vi "CMD_FITLINE.vi"(8 "error in (no error)":errorcluster, 10 "Arguments":string[](array[string]), 11 "gScript Interpreter in":refnum<class "gScript Interpreter.lvclass">) -> (0 "error out":errorcluster, 3 "gScript Interpreter out":refnum<class "gScript Interpreter.lvclass">)   [LabVIEW 2022 SP3, in "gScript Interpreter.lvclass"]
uses:
  gScript Interpreter.lvclass
  gScript Interpreter.lvclass/gScript Interpreter.ctl
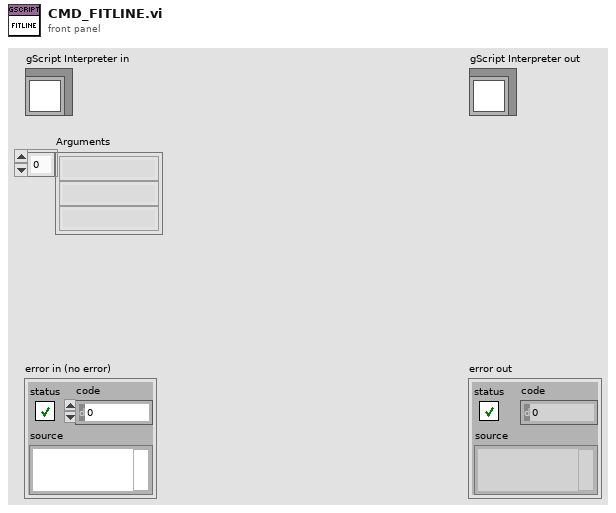
[diagram p1: front panel]
types:
  T1 = typedef "Memory Cell.ctl" = cluster{"type":T2, "x":dbl, "y":dbl, "z":dbl, "w":dbl}
  T2 = typedef "Memory Cell Type Enum.ctl" = enum16{"integer", "float", "vector", "rotation"}
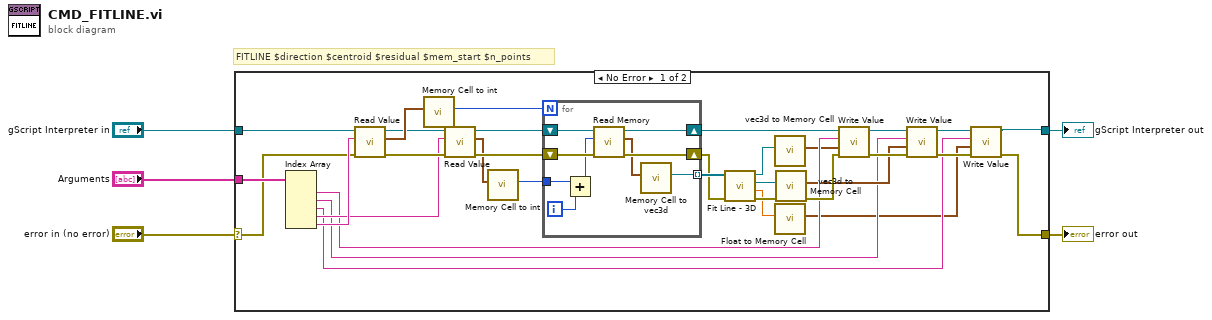
[diagram p0: block diagram]
diagram:
  # "FITLINE $direction $centroid $residual $mem_start $n_points"
  n1 = case shown="No Error" "error in (no error)" {
    selector: "error in (no error)" -> [w34 w48]
    tunnel: [w6 w48] -> w4
    tunnel: [w7 w47] -> w2
    tunnel: "gScript Interpreter in" -> [w36 w47]
    tunnel: "Arguments" -> [w37 _]
    frame No Error {
      n2 = Index Array(array=w37) -> (element #1=w14:string, element #2=w11:string, element #3=w10:string, element #4=w29:string, element #5=w35:string)  [unwired: 5 in]
      n3 = call-dynamic "Read Value.vi"("error in (no error)"=w34, "String in"=w35, "gScript Interpreter in"=w36) -> ("error out"=w30:errorcluster, "Memory Cell"=w33:T1, "gScript Interpreter out"=w31:refnum<class "gScript Interpreter.lvclass">)  [unwired: 6 in]
      n4 = call "Memory Cell to int.vi"("Memory Cell"=w33) -> ("Int out"=w32:i32)  [unwired: 10 in]
      n5 = call-dynamic "Read Value.vi"("error in (no error)"=w30, "String in"=w29, "gScript Interpreter in"=w31) -> ("error out"=w27:errorcluster, "Memory Cell"=w26:T1, "gScript Interpreter out"=w28:refnum<class "gScript Interpreter.lvclass">)  [unwired: 6 in]
      n6 = call "Memory Cell to int.vi"("Memory Cell"=w26) -> ("Int out"=w25:i32)  [unwired: 10 in]
      n7 = for {
        N: w32 -> [_]
        shift-right: [w45] -> w22
        shift-left: w28 -> [w46]
        shift-right: [w43] -> w23
        shift-left: w27 -> [w44]
        tunnel: [w41] -> w24 mode=indexing
        tunnel: w25 -> [w39]
        i -> [w40]
        n8 = Add(x=w39, y=w40) -> (x+y=w38:i32)
        n9 = call-dynamic "Read Memory.vi"("error in (no error)"=w44, "Memory Address"=w38, "gScript Interpreter in"=w46) -> ("error out"=w43:errorcluster, "Memory Cell"=w42:T1, "gScript Interpreter out"=w45:refnum<class "gScript Interpreter.lvclass">)  [unwired: 6 in]
        n10 = call "Memory Cell to vec3d.vi"("Memory Cell"=w42) -> ("Vec3d out"=w41:refnum<class "Vec3d.lvclass">)  [unwired: 10 in]
      }
      n11 = call "Fit Line - 3D.vi"("error in (no error)"=w23, "Points"=w24) -> ("error out"=w19:errorcluster, "residual"=w9:dbl, "centroid"=w15:refnum<class "Vec3d.lvclass">, "direction"=w16:refnum<class "Vec3d.lvclass">)  [unwired: 6 in]
      n12 = call "vec3d to Memory Cell.vi"("Vec3d in"=w16) -> ("Memory Cell"=w13:T1)  [unwired: 10 in]
      n13 = call "Float to Memory Cell.vi"("Float in"=w9) -> ("Memory Cell"=w8:T1)  [unwired: 10 in]
      n14 = call "vec3d to Memory Cell.vi"("Vec3d in"=w15) -> ("Memory Cell"=w12:T1)  [unwired: 10 in]
      n15 = call-dynamic "Write Value.vi"("error in (no error)"=w19, "Value"=w13, "Address"=w14, "gScript Interpreter in"=w22) -> ("error out"=w18:errorcluster, "gScript Interpreter out"=w21:refnum<class "gScript Interpreter.lvclass">)  [unwired: 6 in]
      n16 = call-dynamic "Write Value.vi"("error in (no error)"=w18, "Value"=w12, "Address"=w11, "gScript Interpreter in"=w21) -> ("error out"=w17:errorcluster, "gScript Interpreter out"=w20:refnum<class "gScript Interpreter.lvclass">)  [unwired: 6 in]
      n17 = call-dynamic "Write Value.vi"("error in (no error)"=w17, "Value"=w8, "Address"=w10, "gScript Interpreter in"=w20) -> ("error out"=w6:errorcluster, "gScript Interpreter out"=w7:refnum<class "gScript Interpreter.lvclass">)  [unwired: 6 in]
    }
    frame Error {
    }
  }
  "error out" <- w4
  "gScript Interpreter out" <- w2
